vi "Add Controller.vi"(8 "error in":errorcluster, 10 "Custom Events":refnum<class "Custom Events.lvclass">, 11 "Cell in":refnum<class "Cell.lvclass">) -> (0 "error out":errorcluster, 3 "Cell out":refnum<class "Cell.lvclass">)   [LabVIEW 2024, in "SourceGrid.lvlib" / "Cell.lvclass"]
uses:
  Cell.lvclass
  Controllers/Custom Events/Custom Events.lvclass
  Cell.lvclass/Cell.ctl
  Controllers/Custom Events/Custom Events.lvclass/Custom Events.ctl
  D:/git/Sourcegrid-LabVIEW/dll/SourceGrid.dll
  dll/SourceGrid.dll
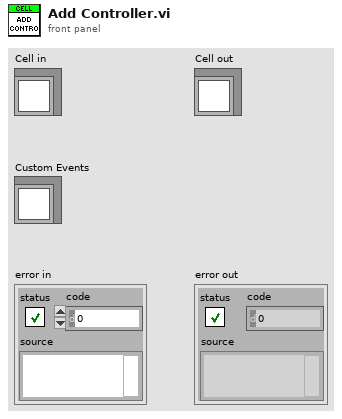
[diagram p1: front panel]
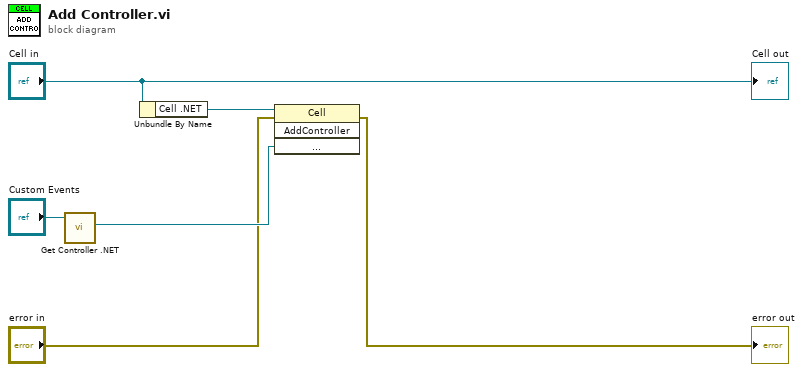
[diagram p0: block diagram]
diagram:
  n1 = call "Get Controller .NET.vi"("Custom Events in"="Custom Events") -> ("Controller .NET"=w3:refnum<k24>)  [unwired: 9 in, 1 out]
  n2 = Unbundle By Name("Cell in") -> ("Cell .NET"=w5:refnum<k24>)
  n3 = invoke class="Cell" method="AddController"(reference=w5, error in="error in", "controller"=w3) -> (error out=→"error out":errorcluster)  [unwired: 1 in, 3 out]
  "Cell out" <- "Cell in"
